vi "casetypescraper.vi"() -> ()   [LabVIEW 2025]
uses:
  <extravilib>/ChannelInstances/Event Messenger-c(str,var).lvlib
  83f7b231-725a-4943-8590-3b7692f63172.vi
  Channel Messages/Bundle Module Message/Bundle Module Message.xnode
  <extravilib>/ChannelInstances/Event Messenger-c(str,var)/))Channel.ctl
panel:
  out "Message Out":T1
  in  "Message In":T1
  in  "Log Text":string
  in  "Log Button":bool
  out "log":string
  in  "module_interface":map{string, variant}(c390)={"Log"=variant(string ""), "Sum"=variant(cluster{"summand0":dbl, "summand1":dbl} {"summand0"=0.0, "summand1"=0.0})}
  out "x+y":dbl
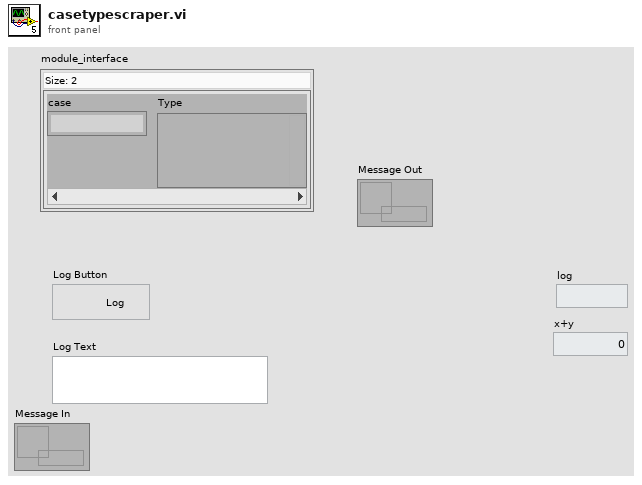
[diagram p1: front panel]
types:
  T1 = typedef "Event Messenger-c(str,var).lvlib/))Channel.ctl" = refnum<queue>
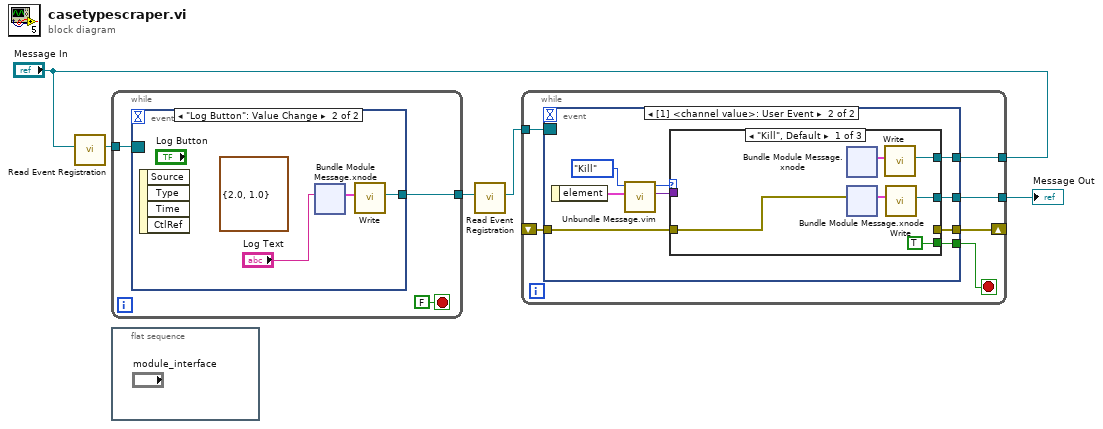
[diagram p0: block diagram]
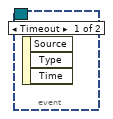
[diagram p2: hidden frame]
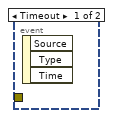
[diagram p3: hidden frame]
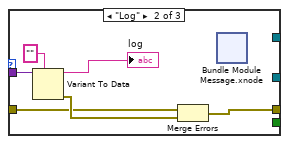
[diagram p4: hidden frame]
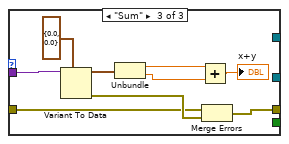
[diagram p5: hidden frame]
diagram:
  n1 = call <extravilib>:"Read Event Registration.vi"("channel"="Message In") -> ("event registration refnum"=w3:refnum<event-registration>)  [unwired: 10 in]
  n2 = while {
    tunnel: [w8] -> w5
    tunnel: w3 -> [w6]
    stop <- FALSE stop-if-true
    n3 = event shown="[1] \"Log Button\": Value Change" {
      selector: w6 -> [_ _]
      dyn-events: _ -> [_ _]
      timeout: _ -> [_ _]
      tunnel: [_ w11] -> w8
      event Timeout {
        n4 = event-data() -> ()  [unwired: 1 in, 3 out]
      }
      event "Log Button": Value Change {
        (unwired) cluster{"summand0":dbl, "summand1":dbl} {"summand0"=2.0, "summand1"=1.0} ("data")
        n5 = event-data() -> ()  [unwired: 1 in, 4 out]
        n6 = xnode "Bundle Module Message.xnode"("data"="Log Text") -> ("message"=w10:cluster{"cmd":string, "data":variant})  [unwired: 1 in, 1 out]
        n7 = call <extravilib>:"Write.vi"("element"=w10) -> ("channel"=w11:T1)  [unwired: 9 in, 1 out]
      }
    }
  }
  n8 = flat-sequence {
    frame #0 {
    }
  }
  n9 = call <extravilib>:"Read Event Registration.vi"("channel"=w5) -> ("event registration refnum"=w4:refnum<event-registration>)  [unwired: 10 in]
  n10 = while {
    tunnel: w4 -> [w22]
    tunnel: "Message In" -> [w19]
    shift-right: [w21] -> _
    shift-left: _ -> [w18]
    tunnel: [w17] -> w1
    stop <- w20 stop-if-true
    n11 = event shown="[1] <channel value>: User Event" {
      selector: w22 -> [_ _]
      dyn-events: _ -> [_ _]
      timeout: _ -> [_ _]
      tunnel: [_ w31] -> w21
      tunnel: [_ w30] -> w20
      tunnel: [_ w25] -> w19
      tunnel: w18 -> [_ w24]
      tunnel: [_ w23] -> w17
      event Timeout {
        n12 = event-data() -> ()  [unwired: 1 in, 3 out]
      }
      event User Event {
        n13 = event-data() -> ("element"=w29:cluster{"cmd":string, "data":variant})  [unwired: 1 in]
        n14 = call "Unbundle Message.vim"("message"=w29, "case type"=enum16{"Kill", "Log", "Sum"}."Kill") -> ("data"=w28:variant, "case"=w27:enum16{"Kill", "Log", "Sum"})  [unwired: 7 in, 1 out]
        n15 = case shown="\"Kill\", Default" w27 {
          tunnel: w28 -> [_ w51 w67]
          tunnel: [_ w49 w60] -> w31
          tunnel: [TRUE _ _] -> w30
          tunnel: [w35 _ _] -> w25
          tunnel: w24 -> [w32 w48 w59]
          tunnel: [w34 _ _] -> w23
          frame "Kill", Default {
            n16 = xnode "Bundle Module Message.xnode"() -> ("message"=w36:cluster{"cmd":string, "data":variant})  [unwired: 2 in, 1 out]
            n17 = xnode "Bundle Module Message.xnode"("data"=w32) -> ("message"=w33:cluster{"cmd":string, "data":variant})  [unwired: 1 in, 1 out]
            n18 = call <extravilib>:"Write.vi"("element"=w36) -> ("channel"=w35:T1)  [unwired: 9 in, 1 out]
            n19 = call <extravilib>:"Write.vi"("element"=w33) -> ("channel"=w34:T1)  [unwired: 9 in, 1 out]
          }
          frame "Log" {
            n20 = Variant To Data(type="", Variant=w51) -> (data=→"log":string, error out=w50:errorcluster)  [unwired: 1 in]
            n21 = Merge Errors(w48, w50) -> (w49:errorcluster)
            n22 = xnode "Bundle Module Message.xnode"() -> ()  [unwired: 2 in, 2 out]
          }
          frame "Sum" {
            n23 = Variant To Data(type=cluster{"summand0":dbl, "summand1":dbl} {"summand0"=0.0, "summand1"=0.0} ("summands"), Variant=w67) -> (data=w65:cluster{"summand0":dbl, "summand1":dbl}, error out=w61:errorcluster)  [unwired: 1 in]
            n24 = Unbundle(w65) -> ("summand0"=w64:dbl, "summand1"=w63:dbl)
            n25 = Add(x=w64, y=w63) -> (x+y=→"x+y":dbl)
            n26 = Merge Errors(w59, w61) -> (w60:errorcluster)
          }
        }
      }
    }
  }
  "Message Out" <- w1
